vi "Check Key Press.vi"(0 "Type":T1, 5 "ScanCode":i16, 7 "Char":i16) -> (4 "Discard?":bool)   [LabVIEW 2015, in "KPropertyTable.xctl"]
uses:
  KPropertyTable.xctl
  DataType.ctl
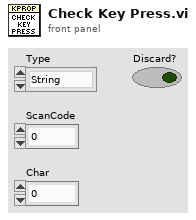
[diagram p1: front panel]
types:
  T1 = typedef "KPropertyTable.xctl/DataType.ctl" = enum16{"String", "Enum", "Int", "Double", "Boolean", "Ring", "Formula"}
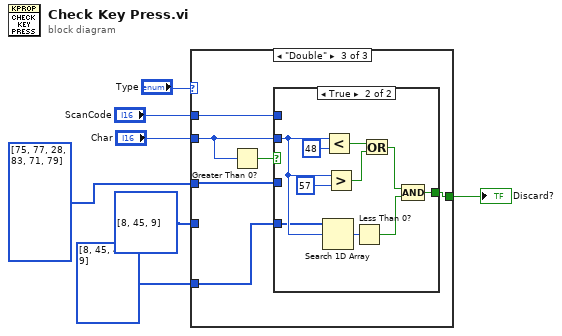
[diagram p0: block diagram]
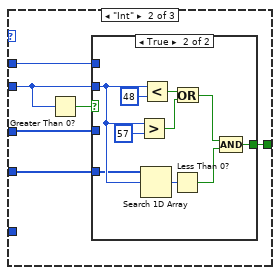
[diagram p3: hidden frame]
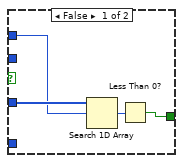
[diagram p4: hidden frame]
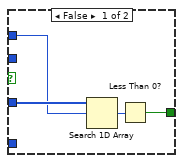
[diagram p5: hidden frame]
diagram:
  n1 = case shown="\"Double\"" "Type" {
    tunnel: "ScanCode" -> [_ w12 w32]
    tunnel: "Char" -> [_ w9 w29]
    tunnel: i32[] [75, 77, 28, 83, 71, 79] -> [_ w11 w31]
    tunnel: [_ w10 w30] -> w3
    tunnel: i32[] [8, 45, 9] -> [_ w8 _]
    tunnel: i32[] [8, 45, 46, 9] -> [_ _ w28]
    frame "String", Default {
    }
    frame "Int" {
      n2 = Greater Than 0?(x=w9) -> (x > 0?=w13:bool)
      n3 = case shown="True" w13 {
        tunnel: w12 -> [w16 _]
        tunnel: w11 -> [w17 _]
        tunnel: [w14 w21] -> w10
        tunnel: w9 -> [_ w24]
        tunnel: w8 -> [_ w23]
        frame False {
          n4 = Search 1D Array(1D array=w17, element=w16) -> (index of element=w15:i32)  [unwired: 1 in]
          n5 = Less Than 0?(x=w15) -> (x < 0?=w14:bool)
        }
        frame True {
          n6 = Greater?(x=w24, y=i16 57) -> (0:w19:bool)
          n7 = Search 1D Array(1D array=w23, element=w24) -> (index of element=w22:i32)  [unwired: 1 in]
          n8 = Less?(x=w24, y=i16 48) -> (x < y?=w25:bool)
          n9 = Less Than 0?(x=w22) -> (x < 0?=w20:bool)
          n10 = Or(x=w25, y=w19) -> (x .or. y?=w18:bool)
          n11 = Compound Arithmetic op=AND(w18, w20) -> (w21:bool)
        }
      }
    }
    frame "Double" {
      n12 = Greater Than 0?(x=w29) -> (x > 0?=w33:bool)
      n13 = case shown="True" w33 {
        tunnel: w32 -> [w36 _]
        tunnel: w31 -> [w37 _]
        tunnel: [w34 w41] -> w30
        tunnel: w29 -> [_ w44]
        tunnel: w28 -> [_ w43]
        frame False {
          n14 = Search 1D Array(1D array=w37, element=w36) -> (index of element=w35:i32)  [unwired: 1 in]
          n15 = Less Than 0?(x=w35) -> (x < 0?=w34:bool)
        }
        frame True {
          n16 = Search 1D Array(1D array=w43, element=w44) -> (index of element=w42:i32)  [unwired: 1 in]
          n17 = Less?(x=w44, y=i16 48) -> (x < y?=w45:bool)
          n18 = Greater?(x=w44, y=i16 57) -> (0:w39:bool)
          n19 = Less Than 0?(x=w42) -> (x < 0?=w40:bool)
          n20 = Or(x=w45, y=w39) -> (x .or. y?=w38:bool)
          n21 = Compound Arithmetic op=AND(w38, w40) -> (w41:bool)
        }
      }
    }
  }
  "Discard?" <- w3
